vi "GLOBAL_baseline.vi"(9 "Addresses In":T1={"TDC"=4026597376, "Scaler"=4026662912, "QDC 1"=4026728448, "QDC 2"=4026793984, "Digitizer 1"=4026859520, "Digitizer 2"=4026925056} {"TDC" format="%.0x"; "Scaler" format="%.0x"; "QDC 1" format="%.0x"; "QDC 2" format="%.0x"; "Digitizer 1" format="%.0x"; "Digitizer 2" format="%.0x"}, 10 "State":enum16{"Initialise", "Write", "Read"}(ring)) -> (1 "Addresses Out":T1={"TDC"=4026597376, "Scaler"=4026662912, "QDC 1"=4026728448, "QDC 2"=4026793984, "Digitizer 1"=4026859520, "Digitizer 2"=4026925056} {"TDC" format="%.0x"; "Scaler" format="%.0x"; "QDC 1" format="%.0x"; "QDC 2" format="%.0x"; "Digitizer 1" format="%.0x"; "Digitizer 2" format="%.0x"})   [LabVIEW 2014]
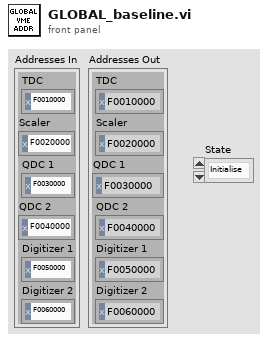
[diagram p1: front panel]
types:
  T1 = cluster{"TDC":u32, "Scaler":u32, "QDC 1":u32, "QDC 2":u32, "Digitizer 1":u32, "Digitizer 2":u32}
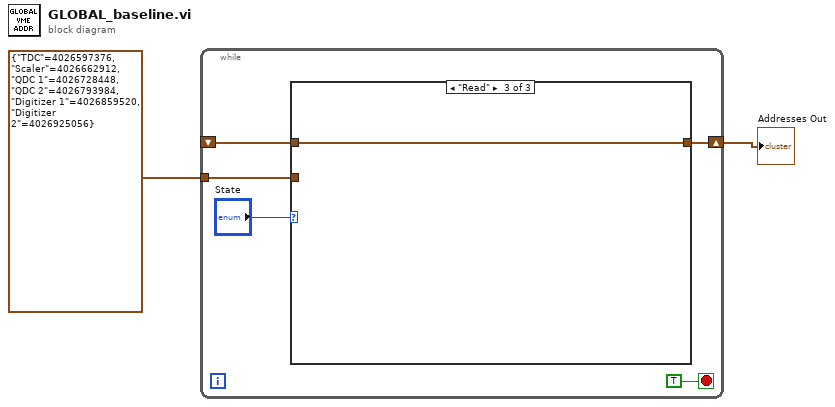
[diagram p0: block diagram]
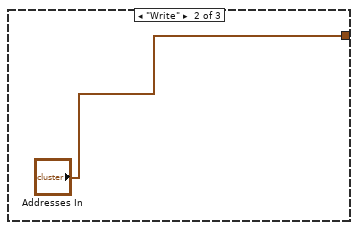
[diagram p3: hidden frame]
diagram:
  n1 = while {
    tunnel: T1 {"TDC"=4026597376, "Scaler"=4026662912, "QDC 1"=4026728448, "QDC 2"=4026793984, "Digitizer 1"=4026859520, "Digitizer 2"=4026925056} -> [w6]
    shift-right: [w5] -> w2
    shift-left: _ -> [w4]
    stop <- TRUE stop-if-true
    n2 = case shown="\"Read\"" "State" {
      tunnel: w6 -> [w8 _ _]
      tunnel: [w8 "Addresses In" w10] -> w5
      tunnel: w4 -> [_ _ w10]
      frame "Initialise", Default {
      }
      frame "Write" {
      }
      frame "Read" {
      }
    }
  }
  "Addresses Out" <- w2
